vi "Orb_Global.vi"() -> ()   [LabVIEW 2009]
panel:
  out "Registered Users":string[](array[string])
  out "Orb Running":bool
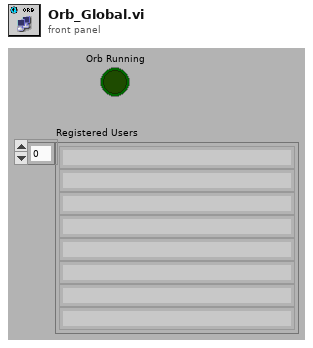
[diagram p1: front panel]
diagram:
